vi "Theme4_Topic1_qn1(SubVI).vi"(9 "RefPrevious":refnum<vi>, 10 "RefNext":refnum<vi>, 11 "connection reference":T1) -> (2 "AnsIndicator":refnum<vi>[](array[refnum]))   [LabVIEW 2013]
uses:
  <vilib>/addons/database/Connection.llb/Conn ObjectReference.ctl
  FYP_LabviewGlobal(SubVI).vi
  <vilib>/addons/database/NI_Database_API.lvlib
panel:
  out "Question":string
  out "Why?":string
  out "DInd":bool
  out "CInd":bool
  out "BInd":bool
  out "AInd":bool
  in  "ABCD":enum32{"No Selection", "A", "B", "C", "D"}(radio)
  out "MCQ_Randomized":string[](array[string])
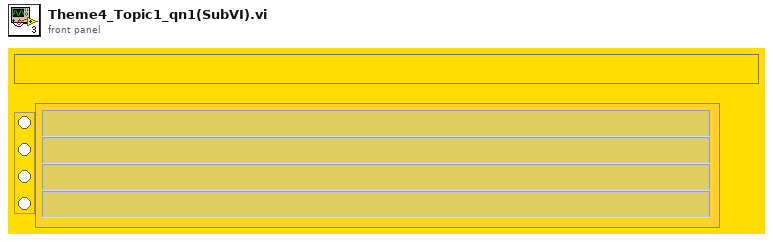
[diagram p1: front panel]
types:
  T1 = typedef "NI_Database_API.lvlib/Conn ObjectReference.ctl" = refnum<k1>
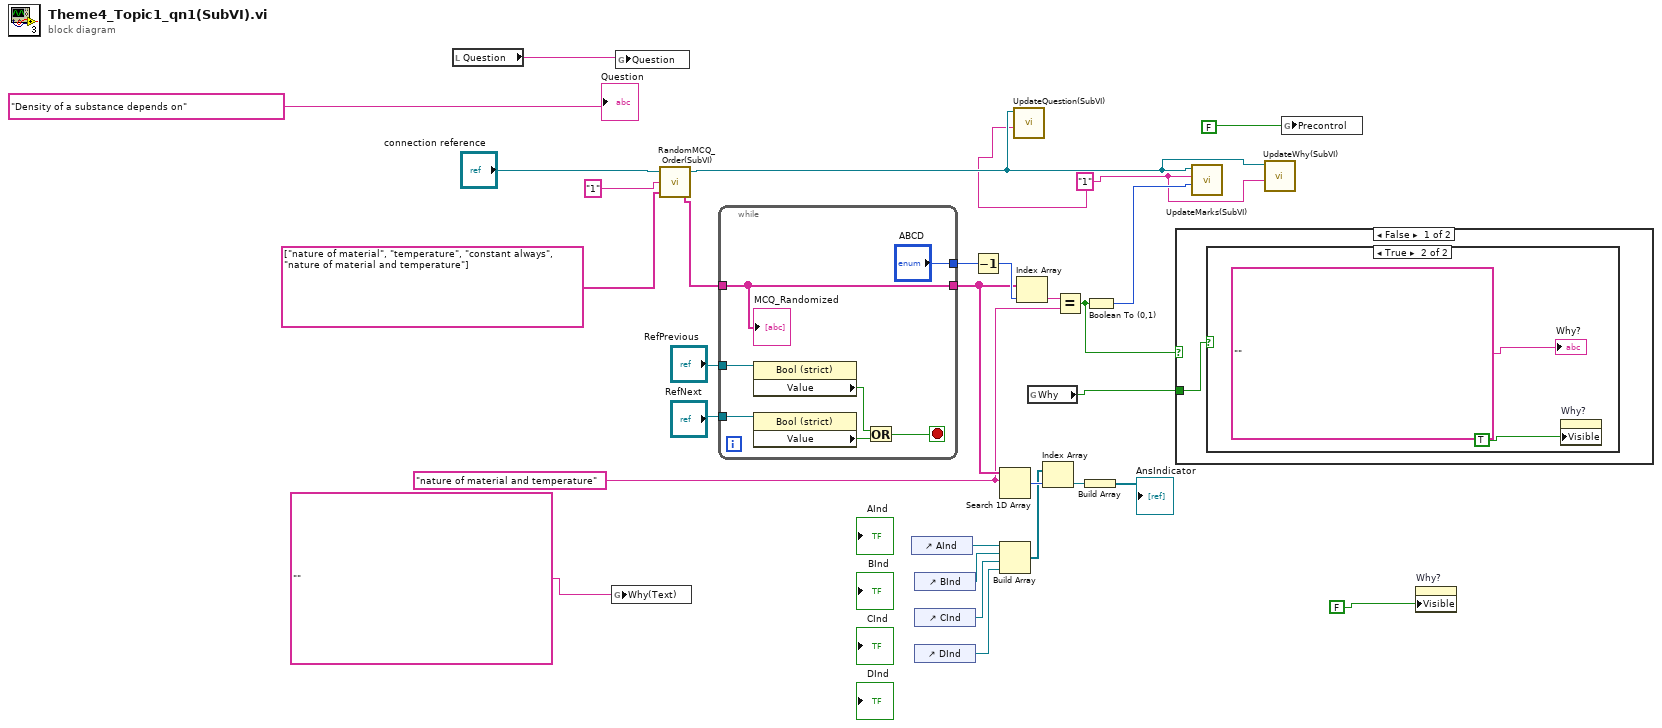
[diagram p0: block diagram]
diagram:
  w2 = "1"
  w18 = "nature of material and temperature" ("element")
  n1 = local read "Question"() -> (w4:string)
  n2 = global write "FYP_LabviewGlobal(SubVI).vi" "Why(Text)"("") -> ()
  n3 = global write "FYP_LabviewGlobal(SubVI).vi" "Question"(w4) -> ()
  n4 = call "RandomMCQ_Order(SubVI).vi"("MCQ_Ordered"=string[] ["nature of material", "temperature", "constant always", "nature of material and temperature"], "Question_Ordered"="1" ("Questions_Ordered"), "connection reference"="connection reference") -> ("MCQ_Randomized"=w11:string[], "connection reference out"=w3:T1)  [unwired: 1 in]
  n5 = while {
    tunnel: ["ABCD"] -> w13
    tunnel: w11 -> [w32]
    tunnel: [w32] -> w20
    tunnel: "RefNext" -> [w33]
    tunnel: "RefPrevious" -> [w34]
    stop <- w31 stop-if-true
    n6 = property class="Bool (strict)"(reference=w34) -> ("Value"=w35:bool)  [unwired: 1 in, 2 out]
    n7 = property class="Bool (strict)"(reference=w33) -> ("Value"=w30:bool)  [unwired: 1 in, 2 out]
    n8 = Or(x=w35, y=w30) -> (x .or. y?=w31:bool)
    "MCQ_Randomized" <- w32
  }
  n9 = control-ref of="AInd"() -> (w27:refnum<vi>)
  n10 = control-ref of="BInd"() -> (w26:refnum<vi>)
  n11 = control-ref of="CInd"() -> (w25:refnum<vi>)
  n12 = control-ref of="DInd"() -> (w24:refnum<vi>)
  n13 = Decrement(x=w13) -> (x-1=w21:enum32{"No Selection", "A", "B", "C", "D"})
  n14 = Search 1D Array(1D array=w20, element=w18) -> (index of element=w23:i32)  [unwired: 1 in]
  n15 = Build Array(w27, w26, w25, w24) -> (w16:refnum<vi>[])
  n16 = call "UpdateQuestion(SubVI).vi"("QuestionsNo_Ordered"=w2, "connection reference"=w3) -> ()  [unwired: 10 in]
  n17 = Index Array(array=w20, index=w21) -> (element=w19:string)
  n18 = global read "FYP_LabviewGlobal(SubVI).vi" "Why"() -> (w12:bool)
  n19 = Index Array(array=w16, index=w23) -> (element=w22:refnum<vi>)
  n20 = Equal?(x=w19, y=w18) -> (x = y?=w14:bool)
  n21 = Build Array(w22) -> (→"AnsIndicator":refnum<vi>[])
  n22 = Boolean To (0,1)(Boolean=w14) -> (0, 1=w9:i16)
  n23 = case shown="False" w14 {
    tunnel: w12 -> [w37 _]
    frame False {
      n24 = case shown="True" w37 {
        frame False {
        }
        frame True {
          n25 = property on="Why?" class="Str"("Visible"=TRUE) -> ()  [unwired: 2 in, 2 out]
          "Why?" <- ""
        }
      }
    }
    frame True {
    }
  }
  n26 = call "UpdateMarks(SubVI).vi"("MarksEarned"=w9, "QuestionsNo_Ordered"=w2, "connection reference"=w3) -> ()  [unwired: 9 in]
  n27 = call "UpdateWhy(SubVI).vi"("QuestionsNo_Ordered"=w2, "connection reference"=w3) -> ()  [unwired: 10 in]
  n28 = global write "FYP_LabviewGlobal(SubVI).vi" "Precontrol"(FALSE) -> ()
  n29 = property on="Why?" class="Str"("Visible"=FALSE) -> ()  [unwired: 2 in, 2 out]
  "Question" <- "Density of a substance depends on"
